vi "Delete Get and SET NO variables from DB.vi"(8 "error in (no error)":errorcluster, 11 "Expt_device_id":string="18") -> (0 "error out":errorcluster)   [LabVIEW 2013]
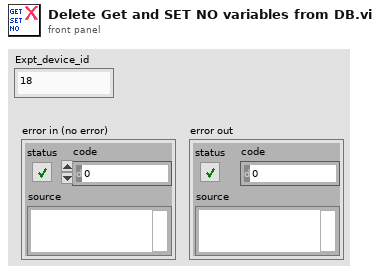
[diagram p1: front panel]
types:
  T1 = typedef "mysql_authentication.ctl" = cluster{"User":string, "Password":string, "Database":string}
  T2 = cluster{"Port":u16, "IP Address":string, "Authentication":T1}
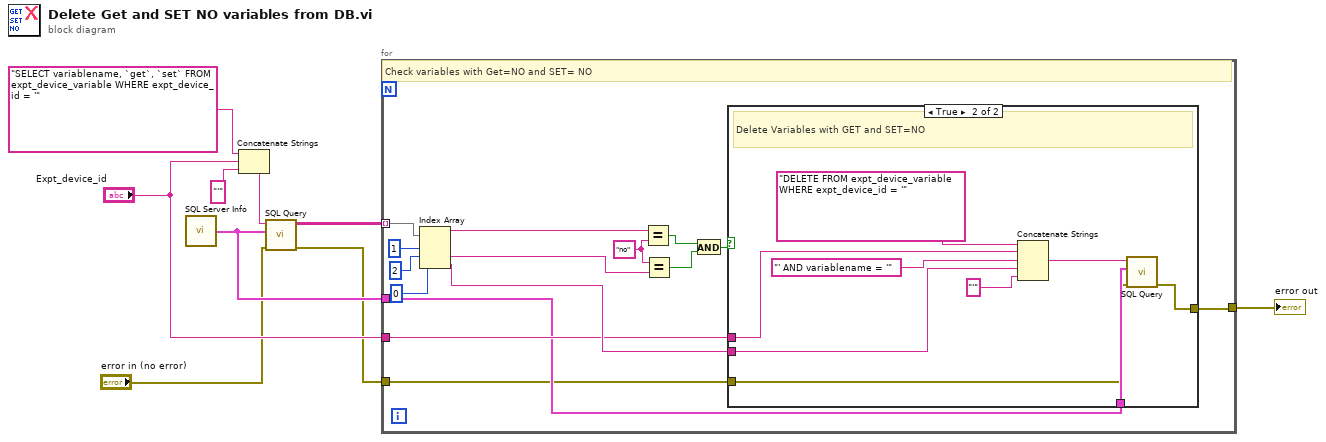
[diagram p0: block diagram]
diagram:
  n1 = call "SQL Server Info.vi"() -> ("SQL Server Info"=w4:T2)
  n2 = Concatenate Strings("SELECT variablename, `get`, `set` FROM expt_device_variable WHERE expt_device_id = '", "Expt_device_id", "'" ("string")) -> (w6:string)
  n3 = call "SQL Query.vi"("error in (no error)"="error in (no error)", "SQL Server Info"=w4, "Query"=w6) -> ("error out"=w2:errorcluster, "data"=w9:string[][])  [unwired: 7 in]
  n4 = for {
    tunnel: w9 -> [w24] mode=indexing
    tunnel: "Expt_device_id" -> [w14]
    tunnel: [w13] -> w3
    tunnel: w4 -> [w12]
    tunnel: w2 -> [w10]
    w19 = "no" ("y")
    # "Check variables with Get=NO and SET= NO"
    n5 = Index Array(array=w24, index #1=1 ("index"), index #2=2 ("index"), index #3=0 ("index")) -> (element #1=w21:string, element #2=w20:string, element #3=w15:string)
    n6 = Equal?(x=w21, y=w19) -> (x = y?=w18:bool)
    n7 = Equal?(x=w19, y=w20) -> (x = y?=w17:bool)
    n8 = And(x=w18, y=w17) -> (x .and. y?=w16:bool)
    n9 = case shown="True" w16 {
      tunnel: w14 -> [_ w29]
      tunnel: w15 -> [_ w28]
      tunnel: [_ w27] -> w13
      tunnel: w12 -> [_ w26]
      tunnel: w10 -> [_ w25]
      frame False {
      }
      frame True {
        # "Delete Variables with GET and SET=NO"
        n10 = Concatenate Strings("DELETE FROM expt_device_variable WHERE expt_device_id = '" ("Query String"), w29, "' AND variablename = '" ("Query String"), w28, "'") -> (w30:string)
        n11 = call "SQL Query.vi"("error in (no error)"=w25, "SQL Server Info"=w26, "Query"=w30) -> ("error out"=w27:errorcluster)  [unwired: 7 in, 1 out]
      }
    }
  }
  "error out" <- w3
